vi "Sys config bundler-Boolean.vi"(7 "Keys setup.Boolean":T2, 8 "error in (no error)":errorcluster, 9 "Section name":string, 10 "System Config to save in":T3={"XY Stage"={"COM port"="", "Baudrate"=0, "Type"=""}, "DAQ FPGA"={"Target"="RIO0", "input card type"=enum."AC Card", "Ref"=refnum, "Clock Freq (MHz) "=200.0, "Samples Wait after Trigger"=5080, "AOD fill"=4900, "StartupDelay"=0, "Slip Cycle (clock cycles)"=600000, "Add Cycle"=TRUE}, "Control system"={"Contrl Sys Available Ind"=FALSE, "Control system.FPGA Type"=enum."Virtex 7", "Control system.Network adapter name"="", "Control system.MAC address"="", "Control system.Ethernet Port"=0, "Ethernet opened"=FALSE, "Ctrl FPGA Clock (MHz)"=240.0, "AOD 1 Amplitude"=0, "AOD 2 Amplitude"=0, "AOD 3 Amplitude"=0, "AOD 4 Amplitude"=0, "AOD 5 Amplitude"=0, "AOD 6 Amplitude"=0, "Data Time Interval (ns)"=0.0, "T0 (ns)"=0.0, "Ta (ns)"=0.0}, "Encoder"={"IP address"="224.0.1.103", "Port"=7000, "Wheel radius (cm)"=16.0, "Encoder Trigger"=""}, "DAQmx Chan"={"Pockels AO"="", "Hard shutter AO"="", "PMT AOs"="", "Galvo AOs"="", "Power meter AI"=""}, "Computer MAC address"="", "Cam VidRec"={"DO flag-Video record"="", "DO flag-Trial start"=""}, "Externalise Triggers"=FALSE, "MC Supported"=FALSE, "Laser wavelength (nm)"=920.0} {"Laser wavelength (nm)" min=800.0 max=1080.0 step=1.0; "Encoder"."Wheel radius (cm)" format="%#_13g"; "Control system"."Control system.Ethernet Port" min=0 max=2048 step=1; "Control system"."Ctrl FPGA Clock (MHz)" min=80.0 max=500.0 step=1.0; "Control system"."Data Time Interval (ns)" min=0.0 max=2048.0 step=1.0; "Control system"."Ta (ns)" min=0.0 max=2048.0 step=1.0; "Control system"."T0 (ns)" min=0.0 max=2048.0 step=1.0; "Control system"."AOD 6 Amplitude" min=0 max=2048 step=1; "Control system"."AOD 5 Amplitude" min=0 max=2048 step=1; "Control system"."AOD 4 Amplitude" min=0 max=2048 step=1; "Control system"."AOD 3 Amplitude" min=0 max=2048 step=1; "Control system"."AOD 2 Amplitude" min=0 max=2048 step=1; "Control system"."AOD 1 Amplitude" min=0 max=2048 step=1}, 11 "Refnum in":T1) -> (0 "error out":errorcluster, 2 "System Config to save":T3={"XY Stage"={"COM port"="", "Baudrate"=0, "Type"=""}, "DAQ FPGA"={"Target"="RIO0", "input card type"=enum."AC Card", "Ref"=refnum, "Clock Freq (MHz) "=200.0, "Samples Wait after Trigger"=5080, "AOD fill"=4900, "StartupDelay"=0, "Slip Cycle (clock cycles)"=600000, "Add Cycle"=TRUE}, "Control system"={"Contrl Sys Available Ind"=FALSE, "Control system.FPGA Type"=enum."Virtex 7", "Control system.Network adapter name"="", "Control system.MAC address"="", "Control system.Ethernet Port"=0, "Ethernet opened"=FALSE, "Ctrl FPGA Clock (MHz)"=240.0, "AOD 1 Amplitude"=0, "AOD 2 Amplitude"=0, "AOD 3 Amplitude"=0, "AOD 4 Amplitude"=0, "AOD 5 Amplitude"=0, "AOD 6 Amplitude"=0, "Data Time Interval (ns)"=0.0, "T0 (ns)"=0.0, "Ta (ns)"=0.0}, "Encoder"={"IP address"="224.0.1.103", "Port"=7000, "Wheel radius (cm)"=16.0, "Encoder Trigger"=""}, "DAQmx Chan"={"Pockels AO"="", "Hard shutter AO"="", "PMT AOs"="", "Galvo AOs"="", "Power meter AI"=""}, "Computer MAC address"="", "Cam VidRec"={"DO flag-Video record"="", "DO flag-Trial start"=""}, "Externalise Triggers"=FALSE, "MC Supported"=FALSE, "Laser wavelength (nm)"=920.0} {"Laser wavelength (nm)" min=800.0 max=1080.0 step=1.0; "Encoder"."Wheel radius (cm)" format="%#_13g"; "Control system"."Control system.Ethernet Port" min=0 max=2048 step=1; "Control system"."Ctrl FPGA Clock (MHz)" min=80.0 max=500.0 step=1.0; "Control system"."Data Time Interval (ns)" min=0.0 max=2048.0 step=1.0; "Control system"."Ta (ns)" min=0.0 max=2048.0 step=1.0; "Control system"."T0 (ns)" min=0.0 max=2048.0 step=1.0; "Control system"."AOD 6 Amplitude" min=0 max=2048 step=1; "Control system"."AOD 5 Amplitude" min=0 max=2048 step=1; "Control system"."AOD 4 Amplitude" min=0 max=2048 step=1; "Control system"."AOD 3 Amplitude" min=0 max=2048 step=1; "Control system"."AOD 2 Amplitude" min=0 max=2048 step=1; "Control system"."AOD 1 Amplitude" min=0 max=2048 step=1}, 3 "Refnum out":T1)   [LabVIEW 2017]
uses:
  Typedefs/XY Stage config cluster.ctl
  <vilib>/userdefined/High Color/nirio_resource_hc.ctl
  RIG-SPECIFIC FILES/FPGA Refs/FPGA Ref.ctl
  Typedefs/FPGA input type AC-DC.ctl
  Typedefs/DAQ FPGA config cluster.ctl
  Typedefs/DAQmx physical channels cluster.ctl
  Typedefs/CTRL system config cluster.ctl
  Typedefs/Encoder config cluster.ctl
  Typedefs/Cam VidRec HW config setup cluster.ctl
  Typedefs/Sys Configuration.ctl
  Typedefs/Ini file interface (Boolean).ctl
  <vilib>/Utility/config.llb/Config Data RefNum.ctl
  <vilib>/Utility/config.llb/NI_LVConfig.lvlib
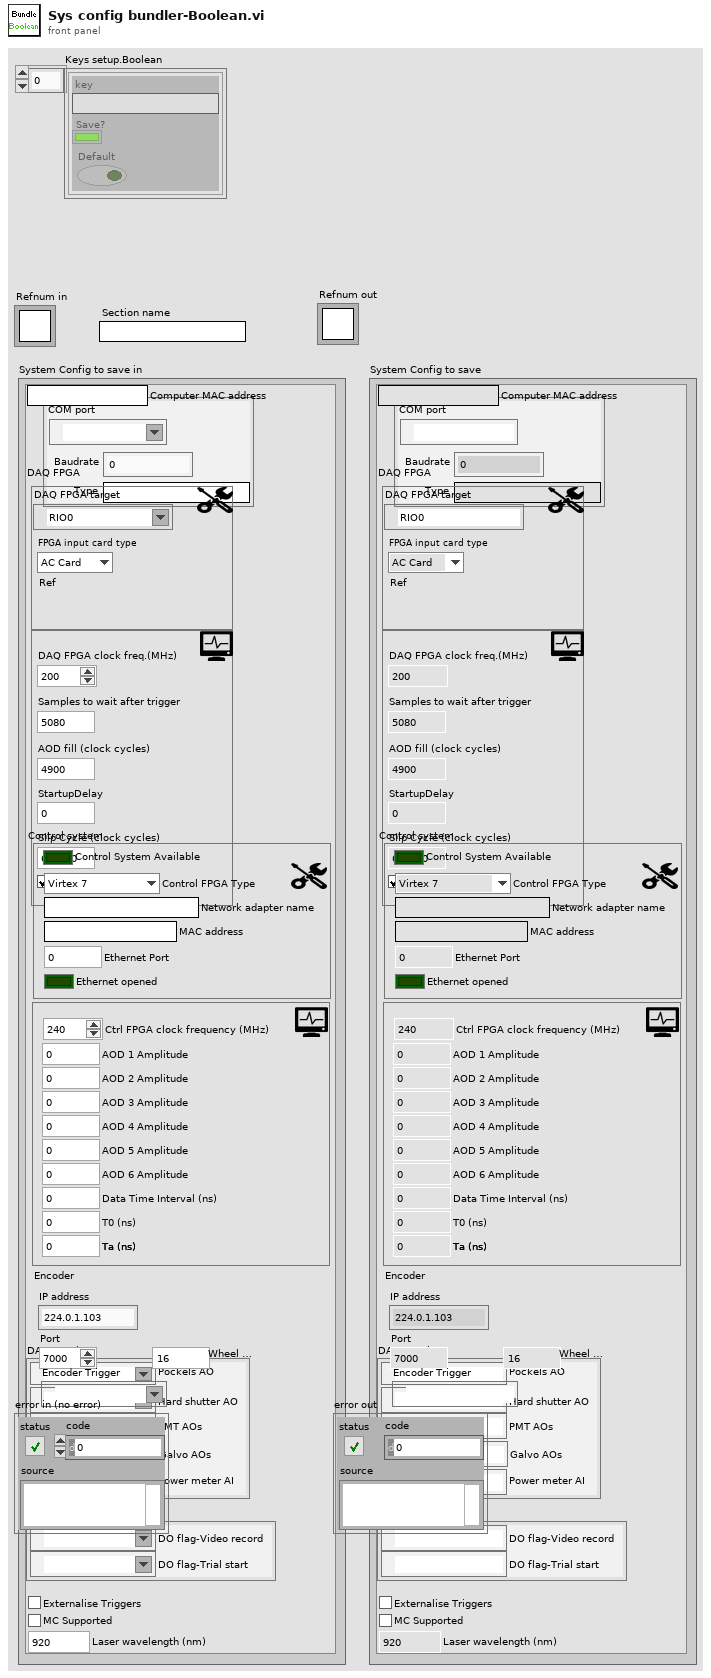
[diagram p1: front panel]
types:
  T1 = typedef "NI_LVConfig.lvlib/Config Data RefNum.ctl" = refnum<k1>
  T2 = typedef "Ini file interface (Boolean).ctl" = cluster{"key":string, "Save?":bool, "Default":bool}[]
  T3 = typedef "Sys Configuration.ctl" = cluster{"XY Stage":T4, "DAQ FPGA":T5, "Control system":T9, "Encoder":T10, "DAQmx Chan":T11, "Computer MAC address":string, "Cam VidRec":T12, "Externalise Triggers":bool, "MC Supported":bool, "Laser wavelength (nm)":dbl}
  T4 = typedef "XY Stage config cluster.ctl" = cluster{"COM port":refnum<visa-resource-name>, "Baudrate":i32, "Type":string}
  T5 = typedef "DAQ FPGA config cluster.ctl" = cluster{"Target":T6, "input card type":T7, "Ref":T8, "Clock Freq (MHz) ":dbl, "Samples Wait after Trigger":u16, "AOD fill":u16, "StartupDelay":i32, "Slip Cycle (clock cycles)":u32, "Add Cycle":bool}
  T6 = typedef "nirio_resource_hc.ctl" = tag
  T7 = typedef "FPGA input type AC-DC.ctl" = enum16{"AC Card", "DC Card"}
  T8 = typedef "FPGA Ref.ctl" = refnum<k20>
  T9 = typedef "CTRL system config cluster.ctl" = cluster{"Contrl Sys Available Ind":bool, "Control system.FPGA Type":enum16{"Virtex 5", "Virtex 7"}, "Control system.Network adapter name":string, "Control system.MAC address":string, "Control system.Ethernet Port":i16, "Ethernet opened":bool, "Ctrl FPGA Clock (MHz)":dbl, "AOD 1 Amplitude":i16, "AOD 2 Amplitude":i16, "AOD 3 Amplitude":i16, "AOD 4 Amplitude":i16, "AOD 5 Amplitude":i16, "AOD 6 Amplitude":i16, "Data Time Interval (ns)":dbl, "T0 (ns)":dbl, "Ta (ns)":dbl}
  T10 = typedef "Encoder config cluster.ctl" = cluster{"IP address":string, "Port":u16, "Wheel radius (cm)":dbl, "Encoder Trigger":tag}
  T11 = typedef "DAQmx physical channels cluster.ctl" = cluster{"Pockels AO":tag, "Hard shutter AO":tag, "PMT AOs":tag, "Galvo AOs":tag, "Power meter AI":tag}
  T12 = typedef "Cam VidRec HW config setup cluster.ctl" = cluster{"DO flag-Video record":tag, "DO flag-Trial start":tag}
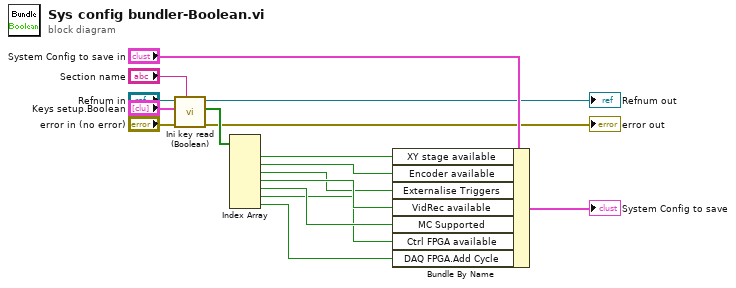
[diagram p0: block diagram]
diagram:
  n1 = call "Ini key read (Boolean).vi"("Section"="Section name", "error in (no error)"="error in (no error)", "Parameter names & setup"="Keys setup.Boolean", "Ini file refnum in"="Refnum in") -> ("error out"=→"error out":errorcluster, "Value read/used"=w9:bool[], "Ini file refnum out"=→"Refnum out":T1)  [unwired: 5 in]
  n2 = Index Array(array=w9) -> (element #1=w12:bool, element #2=w13:bool, element #3=w14:bool, element #4=w15:bool, element #5=w16:bool, element #6=w2:bool, element #7=w1:bool)  [unwired: 7 in]
  n3 = Bundle By Name(cluster="System Config to save in", "XY stage available"=w12, "Encoder available"=w13, "Externalise Triggers"=w14, "VidRec available"=w15, "MC Supported"=w16, "Ctrl FPGA available"=w2, "DAQ FPGA.Add Cycle"=w1) -> (→"System Config to save":T3)
